vi "Desenarea si salvarea unei imagini.vi"() -> ()   [LabVIEW 2024]
uses:
  <vilib>/picture/picture.llb/imagedata.ctl
panel:
  in  "pen 2":T1={"Width"=10, "Style"=enum."Solid"}
  out "new picture":picture
  in  "pen":T1={"Width"=10, "Style"=enum."Solid"}
  in  "stop":bool
  in  "Refresh Button":bool
  in  "image name":string
  in  "Class folder":string
  in  "Save":bool
  out "2D Picture 280x280":picture
  out "image data":T2
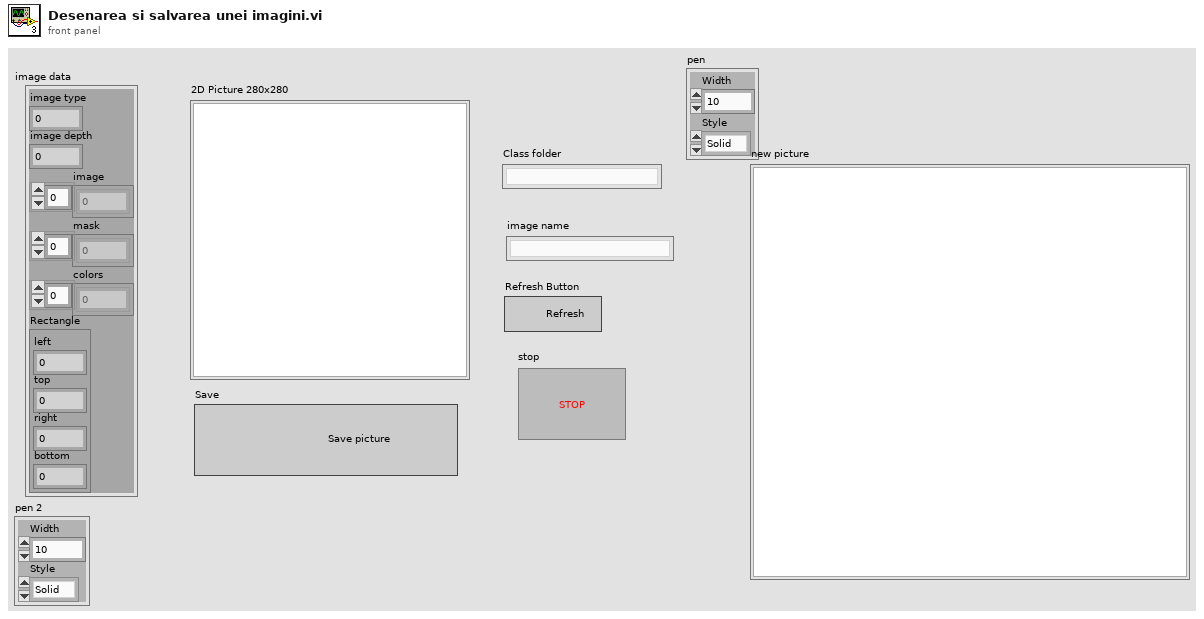
[diagram p1: front panel]
types:
  T1 = cluster{"Width":u16, "Style":enum32{"Solid", "Dash", "Dot", "DashDot", "DashDotDot"}}
  T2 = typedef "imagedata.ctl" = cluster{"image type":i32, "image depth":i32, "image":u8[], "mask":u8[], "colors":u32[], "Rectangle":cluster{"left":i16, "top":i16, "right":i16, "bottom":i16}}
  T3 = cluster{"left":i16, "top":i16, "right":i16, "bottom":i16}
  T4 = typedef "LVMouseTypeDef.ctl" = cluster{"Mouse Position":cluster{"X":i32, "Y":i32}, "Mouse Modifiers":cluster{"Button Down":bool, "Shift Mod":bool, "Menu Mod":bool, "Option Mod":bool}}
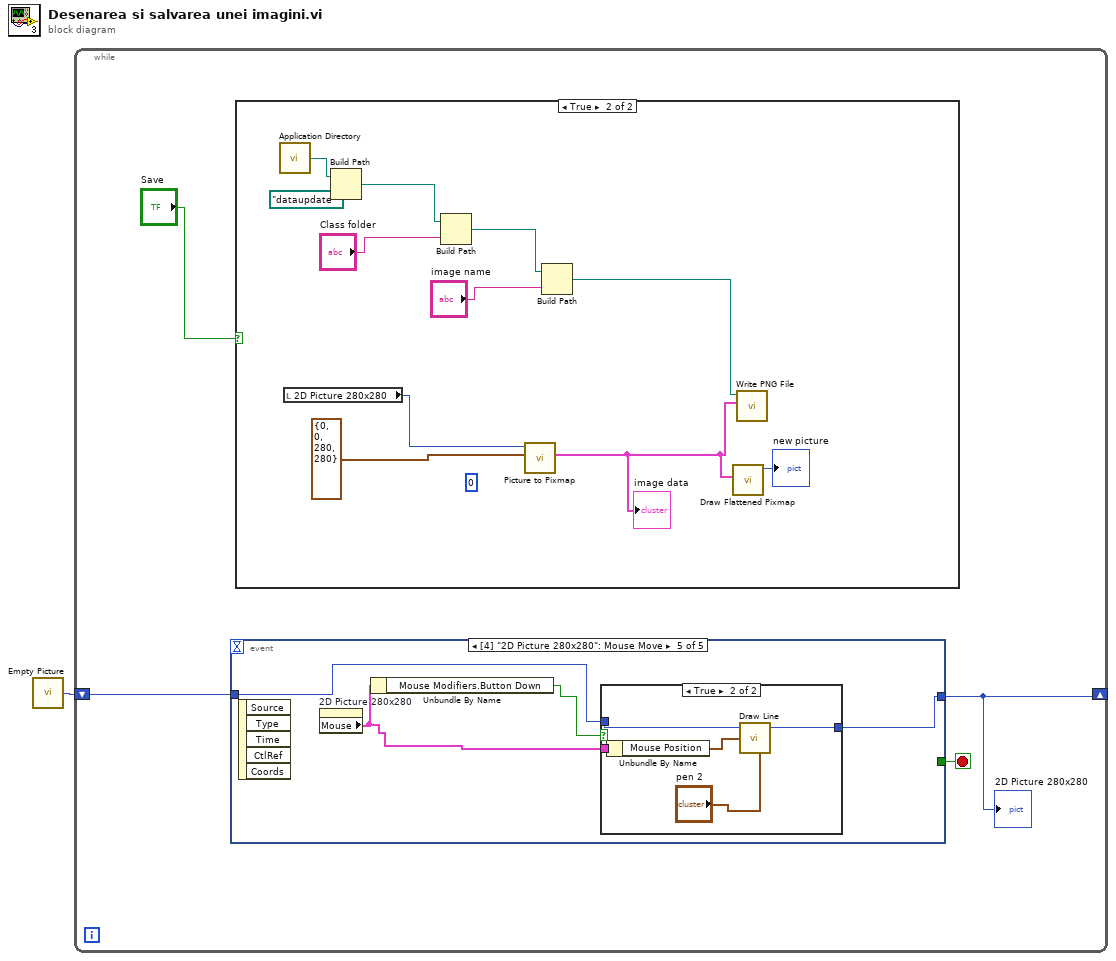
[diagram p0: block diagram]
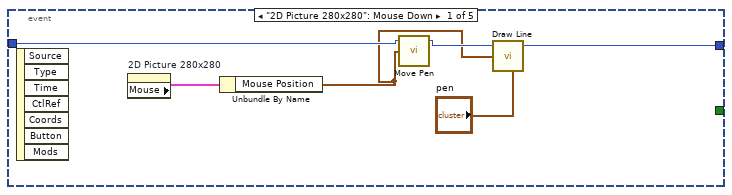
[diagram p2: hidden frame]
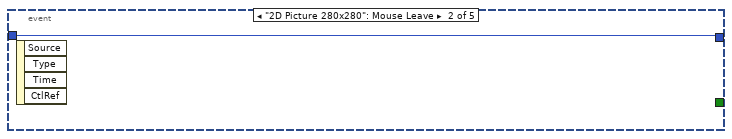
[diagram p3: hidden frame]
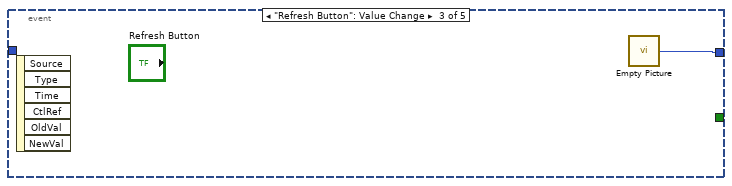
[diagram p4: hidden frame]
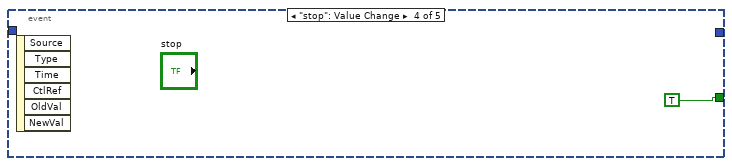
[diagram p5: hidden frame]
diagram:
  n1 = call "Empty Picture"() -> ("empty picture"=w1:picture)
  n2 = while {
    shift-right: [w3] -> _
    shift-left: w1 -> [w4]
    stop <- w2 stop-if-true
    n3 = event shown="[4] \"2D Picture 280x280\": Mouse Move" {
      selector: _ -> [_ _ _ _ _]
      dyn-events: _ -> [_ _ _ _ _]
      timeout: _ -> [_ _ _ _ _]
      tunnel: w4 -> [w10 w12 _ _ w18]
      tunnel: [w6 w12 w13 _ w15] -> w3
      tunnel: [_ _ _ TRUE _] -> w2
      event "2D Picture 280x280": Mouse Down {
        n4 = event-data() -> ()  [unwired: 1 in, 7 out]
        n5 = property on="2D Picture 280x280" class="Pict"() -> ("Mouse"=w11:T4)  [unwired: 2 in, 2 out]
        n6 = Unbundle By Name(w11) -> ("Mouse Position"=w7:cluster{"X":i32, "Y":i32})
        n7 = call <vilib>:"Move Pen.vi"("new position"=w7, "picture"=w10) -> ("new picture"=w9:picture)  [unwired: 3 in]
        n8 = call <vilib>:"Draw Line.vi"("picture"=w9, "end point"=w7, "pen"="pen") -> ("new picture"=w6:picture)  [unwired: 6 in]
      }
      event "2D Picture 280x280": Mouse Leave {
        n9 = event-data() -> ()  [unwired: 1 in, 4 out]
      }
      event "Refresh Button": Value Change {
        n10 = event-data() -> ()  [unwired: 1 in, 6 out]
        n11 = call "Empty Picture"() -> ("empty picture"=w13:picture)
      }
      event "stop": Value Change {
        n12 = event-data() -> ()  [unwired: 1 in, 6 out]
      }
      event "2D Picture 280x280": Mouse Move {
        n13 = event-data() -> ()  [unwired: 1 in, 5 out]
        n14 = property on="2D Picture 280x280" class="Pict"() -> ("Mouse"=w16:T4)  [unwired: 2 in, 2 out]
        n15 = Unbundle By Name(w16) -> ("Mouse Modifiers.Button Down"=w17:bool)
        n16 = case shown="True" w17 {
          tunnel: w18 -> [w19 w23]
          tunnel: w16 -> [_ w24]
          tunnel: [w19 w21] -> w15
          frame False {
          }
          frame True {
            n17 = Unbundle By Name(w24) -> ("Mouse Position"=w22:cluster{"X":i32, "Y":i32})
            n18 = call <vilib>:"Draw Line.vi"("picture"=w23, "end point"=w22, "pen"="pen 2") -> ("new picture"=w21:picture)  [unwired: 6 in]
          }
        }
      }
    }
    "2D Picture 280x280" <- w3
    n19 = case shown="True" "Save" {
      frame False {
      }
      frame True {
        (unwired) 0
        n20 = call <vilib>:"Application Directory.vi"() -> ("Application Directory"=w35:path)
        n21 = local read "2D Picture 280x280"() -> (w29:picture)
        n22 = Build Path(base path=w35, name or relative path=path "dataupdate") -> (appended path=w33:path)
        n23 = Build Path(base path=w33, name or relative path="Class folder") -> (appended path=w31:path)
        n24 = call <vilib>:"Picture to Pixmap.vi"("rect"=T3 {"left"=0, "top"=0, "right"=280, "bottom"=280}, "picture"=w29) -> ("image data"=w26:T2)  [unwired: 8 in, 1 out]
        "image data" <- w26
        n25 = Build Path(base path=w31, name or relative path="image name") -> (appended path=w27:path)
        n26 = call <vilib>:"Draw Flattened Pixmap.vi"("image data"=w26) -> ("new picture"=→"new picture":picture)  [unwired: 8 in]
        n27 = call <vilib>:"Write PNG File.vi"("image data"=w26, "path to PNG file"=w27) -> ()  [unwired: 8 in, 2 out]
      }
    }
  }
